vi "initGeneralStop.vi"   [LabVIEW 2017]
uses:
  globalUtilities.vi
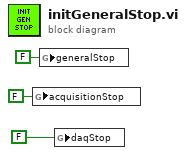
[diagram p0: block diagram]
diagram:
  n1 = global write "globalUtilities.vi" "acquisitionStop"(FALSE ("generalStop")) -> ()
  n2 = global write "globalUtilities.vi" "generalStop"(FALSE ("generalStop")) -> ()
  n3 = global write "globalUtilities.vi" "daqStop"(FALSE ("acquisitionStop")) -> ()
